vi "Reset Analysis ROI.vi"(8 "error in (no error)":errorcluster, 11 "Analysis Graph in":refnum<class "Analysis Graph.lvclass">) -> (0 "error out":errorcluster, 3 "Analysis Graph out":refnum<class "Analysis Graph.lvclass">)   [LabVIEW 2023, in "Analysis Graph.lvclass"]
uses:
  Analysis Graph.lvclass
  Analysis Graph.lvclass/Analysis Graph.ctl
  Detail Graph/Detail Graph.lvclass
  Series Graph/Series Graph.lvclass
  D:/git/Graph-Classes/Series Graph/Series Graph.lvclass
  D:/git/Graph-Classes/Detail Graph/Detail Graph.lvclass
  D:/git/Graph-Classes/Base Graph/Base Graph.lvclass
  D:/git/Graph-Classes/Analysis Graph/Analysis Graph.lvclass
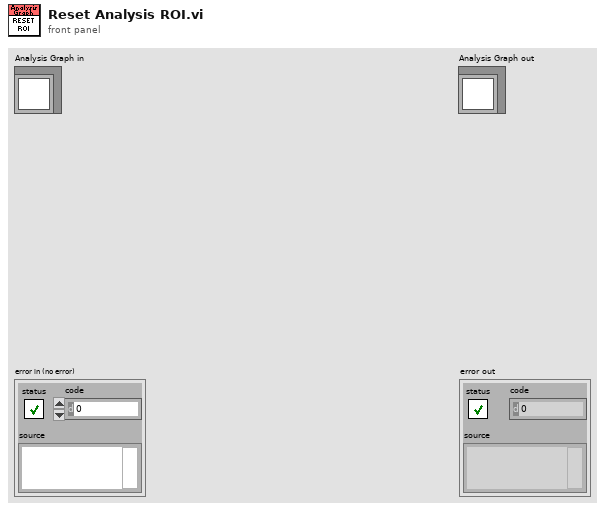
[diagram p1: front panel]
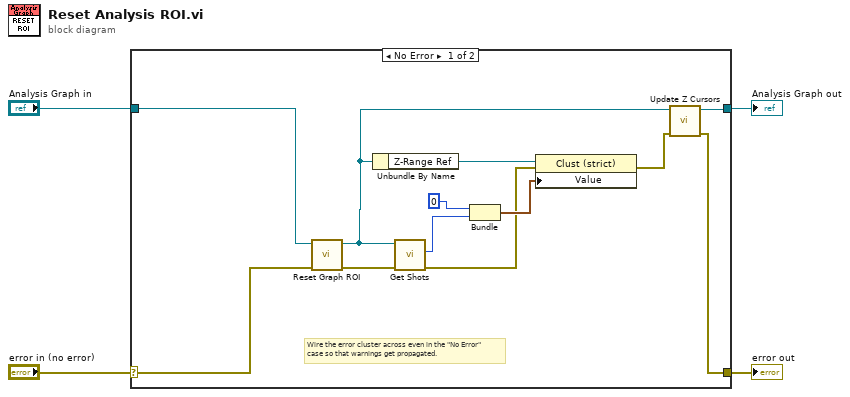
[diagram p0: block diagram]
diagram:
  n1 = case shown="No Error" "error in (no error)" {
    selector: "error in (no error)" -> [w15 w18]
    tunnel: [w6 w18] -> w3
    tunnel: [w5 w17] -> w1
    tunnel: "Analysis Graph in" -> [w16 w17]
    frame No Error {
      # "Wire the error cluster across even in the \"No Error\"\ncase so that warnings get propagated."
      n2 = call "Reset Graph ROI.vi"("error in (no error)"=w15, "Detail Graph. in"=w16) -> ("error out"=w10:errorcluster, "Detail Graph. out"=w8:refnum<class "Analysis Graph.lvclass">)  [unwired: 8 in]
      n3 = Unbundle By Name(w8) -> ("Z-Range Ref"=w14:refnum<vi>)
      n4 = call "Get Shots.vi"("error in (no error)"=w10, "Series Graph in"=w8) -> ("error out"=w9:errorcluster, "Shots"=w13:u32)  [unwired: 7 in, 1 out]
      n5 = Bundle(0, "Shots"=w13) -> (w11:cluster{i32, "Shots":u32})  [unwired: 1 in]
      n6 = property class="Clust (strict)"(reference=w14, error in=w9, "Value"=w11) -> (error out=w7:errorcluster)  [unwired: 1 out]
      n7 = call "Update Z Cursors.vi"("error in (no error)"=w7, "Analysis Graph in"=w8) -> ("error out"=w6:errorcluster, "Analysis Graph out"=w5:refnum<class "Analysis Graph.lvclass">)  [unwired: 8 in]
    }
    frame Error {
    }
  }
  "error out" <- w3
  "Analysis Graph out" <- w1
